vi "Example 1 - Local Bus DBL.vi"() -> ()   [LabVIEW 2021]
uses:
  Omni-Bus/Omni_Bus.lvclass
  Omni-Bus/Support/Broad Types.ctl
  Local Bus/Local Bus.lvclass
  C:/Users/Tim/Documents/GitHub/Omni-Bus/Source/Omni-Bus/Bus Access/Bus_Access.lvclass
  <vilib>/Utility/Data Type/Type Definitions/Data Type.ctl
  Omni-Bus/Support/Read/Read DBL.vi
  <vilib>/TSA/Abstract Data Classes/Abs_Types/Double Float/Abs_Double Float.lvclass
  Omni-Bus/Support/Write/Write DBL.vi
  <vilib>/Utility/Data Type/NI_Data Type.lvlib
panel:
  out "Read error":errorcluster
  out "Write error":errorcluster
  in  "Write Numeric":dbl
  in  "Write Tag":string
  in  "stop":bool
  out "Read Numeric":dbl format="%.2f"
  in  "Read Tag":string
  out "error out":errorcluster
  out "All Tags":string[](array[string])
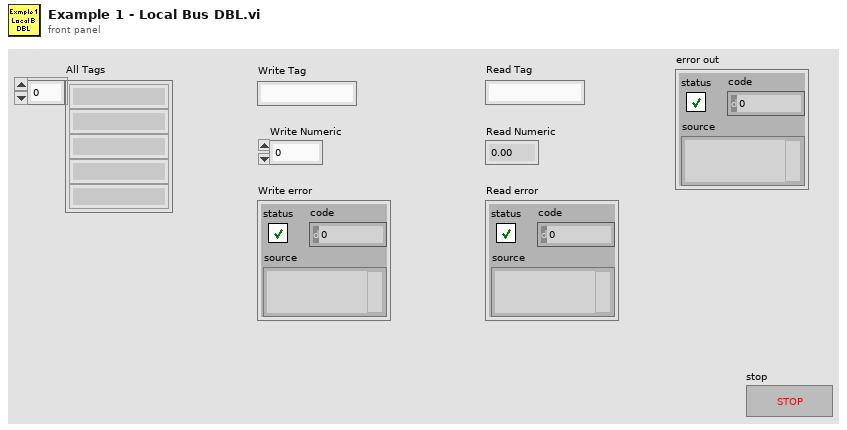
[diagram p1: front panel]
types:
  T1 = typedef "NI_Data Type.lvlib/Data Type.ctl" = enum8{"Invalid Type", "Void", "I8", "I16", "I32", "I64", "U8", "U16", "U32", "U64", "Single Float", "Double Float", "Extended Float", "Single Complex", "Double Complex", "Extended Complex", "Enum U8", "Enum U16", "Enum U32", "Enum U64", "Single Float With Unit", "Double Float With Unit", "Extended Float With Unit", "Single Complex with Unit", "Double Complex with Unit", "Extended Complex with Unit", "Boolean", "String", "Path", "Picture", "Tag", "Array", "Cluster", "Variant", "LV Variant", "Waveform", "Timestamp", "Digital Waveform", "Digital Data", "ExpressData", "Refnum", "External Data", "VI", "Poly VI", "LabVIEW Class Instance", "Fixed Point", "Set Collection", "Map Collection"}
  T2 = typedef "Omni_Bus.lvclass/Broad Types.ctl" = enum16{"All Tags", "NI Specific Type", "Boolean", "String", "Numeric", "Float", "Integer", "Collection", "All Value Types", "Non Value Types"}
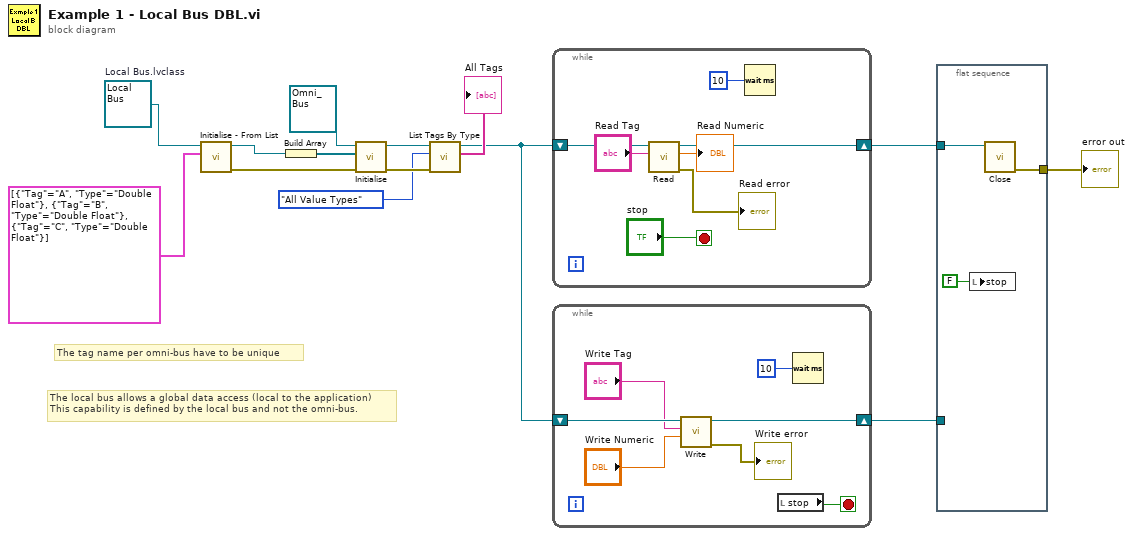
[diagram p0: block diagram]
diagram:
  w2 = refnum<class "Local Bus.lvclass"> refnum  # Local Bus.lvclass
  # "The local bus allows a global data access (local to the application)\nThis capability is defined by the local bus and not the omni-bus."
  # "The tag name per omni-bus have to be unique"
  n1 = call "Initialise - From List.vi"("Tag List"=cluster{"Tag":string, "Type":T1}[] [{"Tag"="A", "Type"=enum."Double Float"}, {"Tag"="B", "Type"=enum."Double Float"}, {"Tag"="C", "Type"=enum."Double Float"}], "Local Bus in"=w2) -> ("error out"=w4:errorcluster, "Local Bus out"=w3:refnum<class "Local Bus.lvclass">)  [unwired: 8 in]
  n2 = Build Array(w3) -> (w13:refnum<class "Local Bus.lvclass">[])
  n3 = call-dynamic "Initialise.vi"("error in (no error)"=w4, "Bus Access"=w13, "Var Bus in"=refnum<class "Omni_Bus.lvclass"> refnum) -> ("error out"=w11:errorcluster, "Var Bus out"=w12:refnum<class "Omni_Bus.lvclass">)  [unwired: 7 in]
  n4 = call-dynamic "List Tags By Type.vi"("error in (no error)"=w11, "Broad Types"=Broad_Types."All Value Types", "Var Bus in"=w12) -> ("Tags"=→"All Tags":string[], "Var Bus out"=w6:refnum<class "Omni_Bus.lvclass">)  [unwired: 5 in, 2 out]
  n5 = while {
    shift-right: [w20] -> w7
    shift-left: w6 -> [w21]
    stop <- "stop" stop-if-true
    n6 = call-poly "Read.vi"("Tag"="Read Tag", "Var Bus in"=w21) -> ("error out"=→"Read error":errorcluster, "Numeric"=→"Read Numeric":dbl, "Var Bus out"=w20:refnum<class "Omni_Bus.lvclass">)  [unwired: 7 in]
    n7 = Wait (ms)(milliseconds to wait=u32 10) -> ()  [unwired: 1 out]
  }
  n8 = while {
    shift-right: [w27] -> w5
    shift-left: w6 -> [w28]
    stop <- w24 stop-if-true
    n9 = call-poly "Write.vi"("Numeric"="Write Numeric", "Tag"="Write Tag", "Omni_Bus in"=w28) -> ("error out"=→"Write error":errorcluster, "Omni_Bus out"=w27:refnum<class "Omni_Bus.lvclass">)  [unwired: 7 in]
    n10 = local read "stop"() -> (w24:bool)
    n11 = Wait (ms)(milliseconds to wait=u32 10) -> ()  [unwired: 1 out]
  }
  n12 = flat-sequence {
    tunnel: [w31] -> w8
    tunnel: w7 -> [w30]
    tunnel: w5 -> [_]
    frame #0 {
      n13 = local write "stop"(FALSE ("stop")) -> ()
      n14 = call-dynamic "Close.vi"("Data in"=w30) -> ("error out"=w31:errorcluster)  [unwired: 9 in, 1 out]
    }
  }
  "error out" <- w8
